vi "WriteTimestampAndFrameIdx.vi"(0 "object in":refnum<class "TDMSLogger.lvclass">, 5 "error in (no error)":errorcluster) -> (14 "object out":refnum<class "TDMSLogger.lvclass">, 19 "error out":errorcluster)   [LabVIEW 2023, in "TDMSLogger.lvclass"]
uses:
  TDMSLogger.lvclass
  TDMSLogger.lvclass/TDMSLogger.ctl
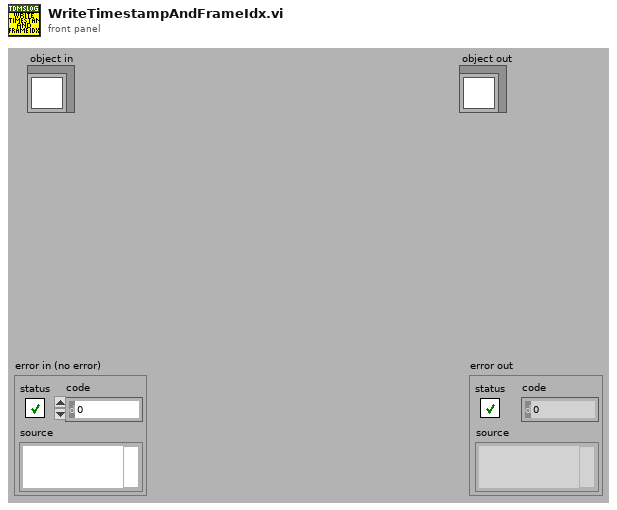
[diagram p1: front panel]
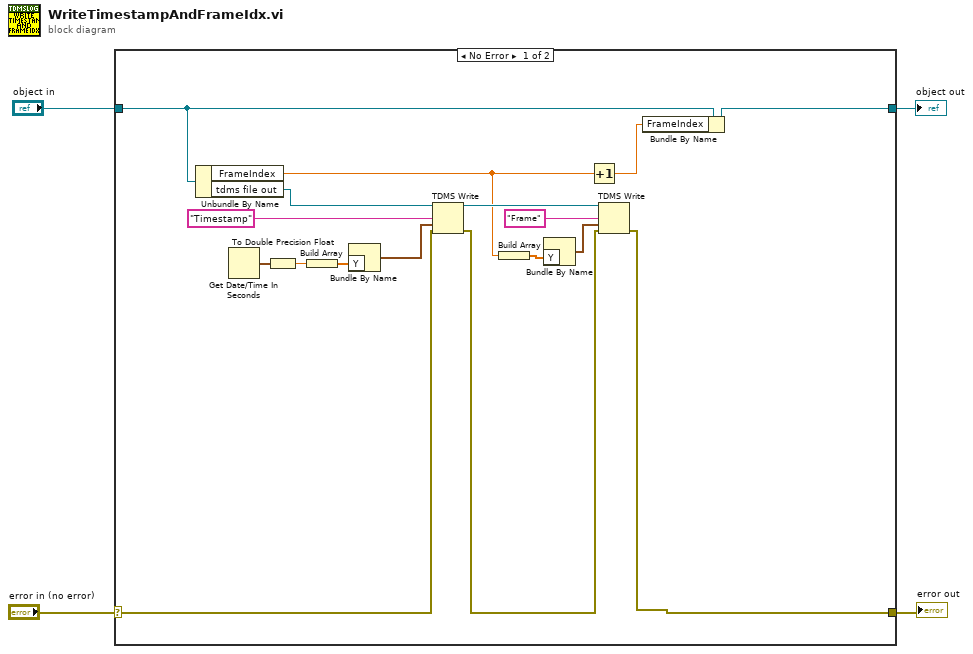
[diagram p0: block diagram]
diagram:
  n1 = case shown="No Error" "error in (no error)" {
    selector: "error in (no error)" -> [w14 w23]
    tunnel: [w6 w23] -> w3
    tunnel: [w9 w22] -> w1
    tunnel: "object in" -> [w21 w22]
    frame No Error {
      n2 = Unbundle By Name(w21) -> ("FrameIndex"=w10:dbl, "tdms file out"=w15:refnum<k34>)
      n3 = Get Date/Time In Seconds() -> (seconds since 1Jan1904=w20:timestamp)
      n4 = To Double Precision Float(number=w20) -> (double precision float=w19:dbl)
      n5 = Build Array(w19) -> (w18:dbl[])
      n6 = Bundle By Name("Y"=w18) -> (w17:waveform(dbl))  [unwired: 1 in]
      n7 = TDMS Write(0:w15, 7:"Timestamp" ("channel name(s) in (Untitled)"), 9:w17, 11:w14) -> (4:w13:refnum<k34>, 15:w7:errorcluster)  [unwired: 2 in, 2 out]
      n8 = Build Array(w10) -> (w12:dbl[])
      n9 = Bundle By Name("Y"=w12) -> (w11:waveform(dbl))  [unwired: 1 in]
      n10 = Increment(x=w10) -> (x+1=w8:dbl)
      n11 = TDMS Write(0:w13, 7:"Frame" ("channel name(s) in (Untitled)"), 9:w11, 11:w7) -> (15:w6:errorcluster)  [unwired: 2 in, 3 out]
      n12 = Bundle By Name(cluster=w21, "FrameIndex"=w8) -> (w9:refnum<class "TDMSLogger.lvclass">)
    }
    frame Error {
    }
  }
  "error out" <- w3
  "object out" <- w1
